vi "KnifeEdge_SimulationSignal_generation_test.vi"() -> ()   [LabVIEW 2012]
uses:
  <vilib>/gmath/SpecialFunctions.llb/Error Function.vi
panel:
  out "Waveform Graph":dbl[](graph)
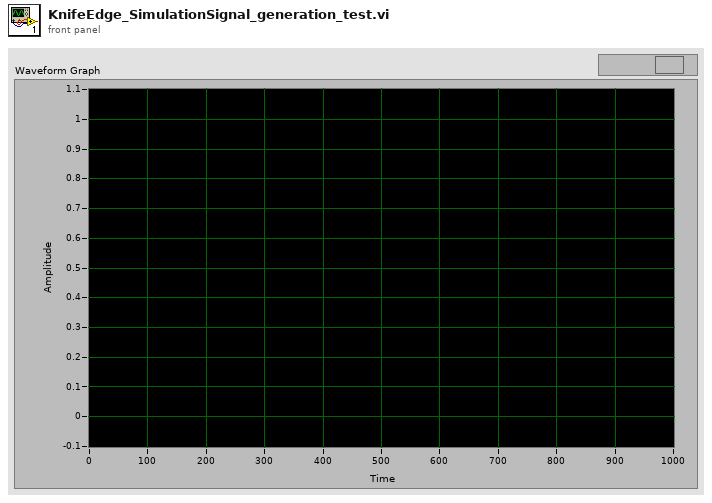
[diagram p1: front panel]
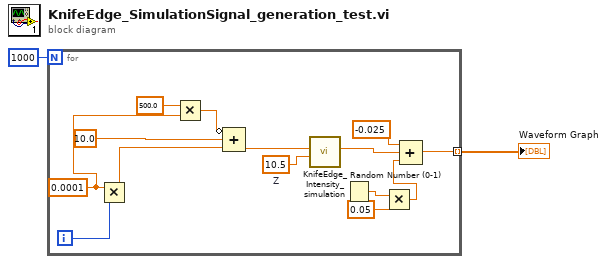
[diagram p0: block diagram]
diagram:
  n1 = for {
    N: 1000 -> [_]
    tunnel: [w12] -> w1 mode=indexing
    i -> [w16]
    w14 = 10.5  # Z
    w5 = 0.0001 ("x")
    n2 = Multiply(x=w5, y=w16) -> (x*y=w15:dbl)
    n3 = Multiply(x=500.0, y=w5) -> (x*y=w3:dbl)
    n4 = Compound Arithmetic op=ADD(invert w3, 10.0 ("x"), w15) -> (w7:dbl)
    n5 = call "KnifeEdge_Intensity_simulation.vi"("Z"=w14, "X"=w7) -> ("E"=w13:dbl)  [unwired: 9 in]
    n6 = Random Number (0-1)() -> (number: 0 to 1=w11:dbl)
    n7 = Multiply(x=w11, y=0.05) -> (x*y=w8:dbl)
    n8 = Compound Arithmetic op=ADD(-0.025 ("value"), w13, w8) -> (w12:dbl)
  }
  "Waveform Graph" <- w1
